vi "Tx End.vi"(8 "error in":errorcluster, 11 "framework in":refnum<class "Framework.lvclass">) -> (0 "error out":errorcluster, 3 "framework out":refnum<class "Framework.lvclass">)   [LabVIEW 2019, in "DSF Core.lvlib" / "Framework.lvclass"]
uses:
  Framework.lvclass
  Framework.lvclass/Framework.ctl
  Performance/Performance.lvclass/Performance.ctl
  Performance/Performance.lvclass
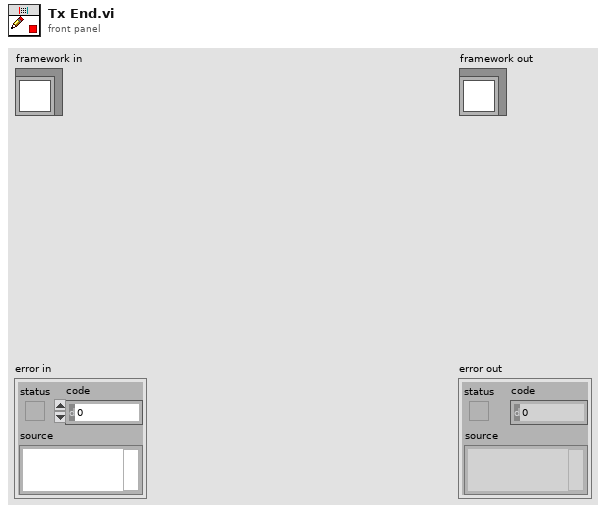
[diagram p1: front panel]
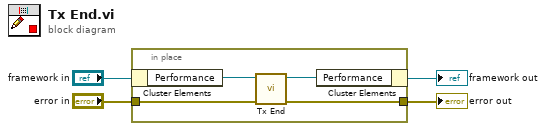
[diagram p0: block diagram]
diagram:
  n1 = in-place {
    in-place-border: "error in" -> [w6]
    in-place-border: [w5] -> w2
    n2 = in-place-cluster #1("framework in") -> ("Performance"=w8:refnum<class "Performance.lvclass">)
    n3 = call "Tx End.vi"("error in"=w6, "performance in"=w8) -> ("error out"=w5:errorcluster, "performance out"=w7:refnum<class "Performance.lvclass">)  [unwired: 8 in]
    n4 = in-place-cluster #1("Performance"=w7) -> (→"framework out":refnum<class "Framework.lvclass">)
  }
  "error out" <- w2
